vi "UpdateHawkeyeList.vi"(7 "WorkSpace / Repo path":path, 8 "error in (no error)":errorcluster, 10 "Library/Class Name":string, 11 "Config Refnum in":T1) -> (0 "error out":errorcluster, 1 "Indirect Dependency []":string[](array[string]), 2 "Direct Dependency []":string[](array[string]), 3 "Config Refnum out":T1)   [LabVIEW 2019, in "Hawkeye.lvlib"]
uses:
  Hawkeye.lvlib
  <vilib>/Utility/config.llb/Config Data RefNum.ctl
  <vilib>/Utility/config.llb/Write Key (String).vi
  <vilib>/Utility/config.llb/NI_LVConfig.lvlib
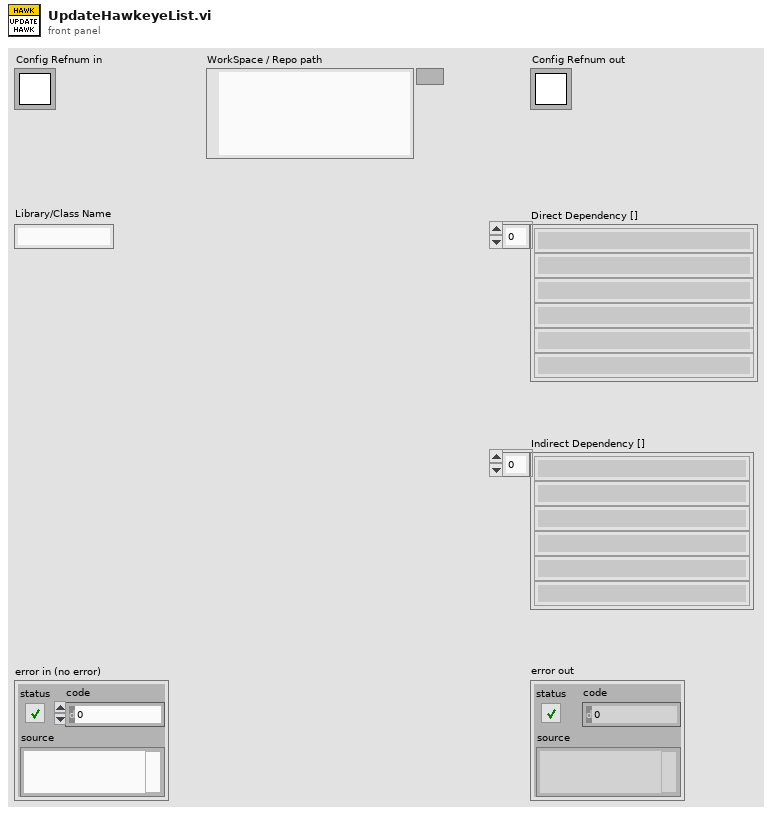
[diagram p1: front panel]
types:
  T1 = typedef "NI_LVConfig.lvlib/Config Data RefNum.ctl" = refnum<k1>
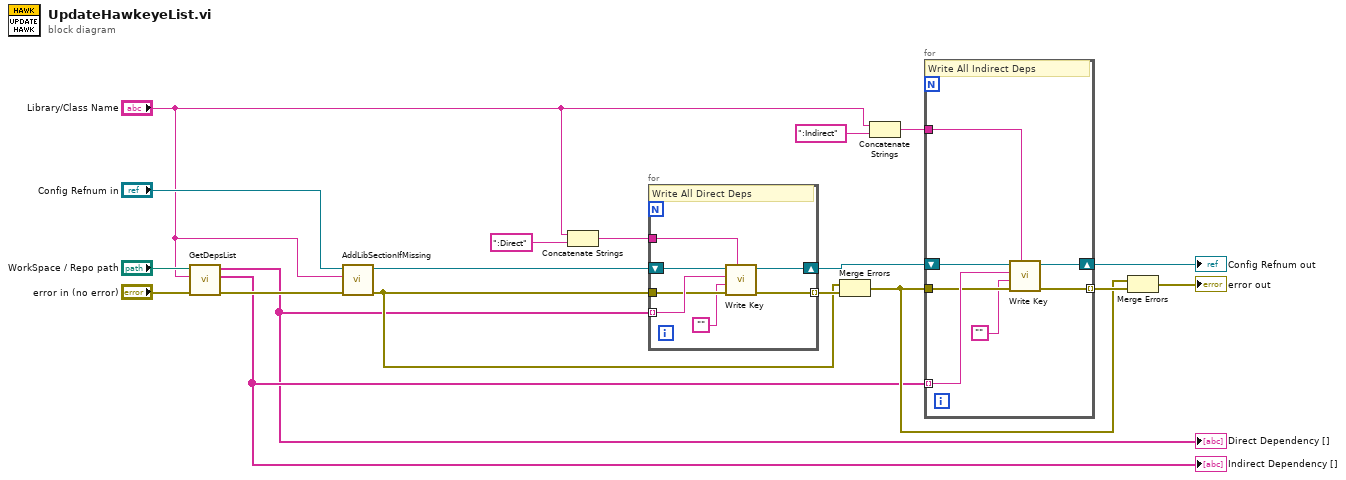
[diagram p0: block diagram]
diagram:
  n1 = call "GetDepsList.vi"("error in (no error)"="error in (no error)", "Library / Class Name"="Library/Class Name", "WorkSpace / Repo path"="WorkSpace / Repo path") -> ("error out"=w6:errorcluster, "Indirect Dependency []"=w2:string[], "Direct Dependency []"=w1:string[])  [unwired: 6 in]
  "Direct Dependency []" <- w1
  "Indirect Dependency []" <- w2
  n2 = call "AddLibSectionIfMissing.vi"("error in (no error)"=w6, "LibraryName"="Library/Class Name", "Config Refnum in"="Config Refnum in") -> ("error out"=w12:errorcluster, "Config Refnum out"=w14:T1)  [unwired: 7 in]
  n3 = Concatenate Strings("Library/Class Name", ":Direct" ("Type")) -> (w15:string)
  n4 = for {
    tunnel: w15 -> [w26]
    tunnel: w1 -> [w24] mode=indexing
    shift-right: [w23] -> w8
    shift-left: w14 -> [w25]
    tunnel: w12 -> [w22]
    tunnel: [w21] -> w13 mode=indexing
    # "Write All Direct Deps"
    n5 = call-poly <vilib>:"Write Key.vi"("section"=w26, "error in (no error)"=w22, "value"="", "key"=w24, "refnum"=w25) -> ("error out"=w21:errorcluster, "refnum out"=w23:T1)  [unwired: 4 in, 1 out]
  }
  n6 = Merge Errors(w12, w13) -> (w10:errorcluster)
  n7 = Concatenate Strings("Library/Class Name", ":Indirect" ("Type")) -> (w9:string)
  n8 = for {
    tunnel: w9 -> [w33]
    tunnel: w2 -> [w31] mode=indexing
    shift-right: [w30] -> w7
    shift-left: w8 -> [w32]
    tunnel: w10 -> [w29]
    tunnel: [w28] -> w11 mode=indexing
    # "Write All Indirect Deps"
    n9 = call-poly <vilib>:"Write Key.vi"("section"=w33, "error in (no error)"=w29, "value"="", "key"=w31, "refnum"=w32) -> ("error out"=w28:errorcluster, "refnum out"=w30:T1)  [unwired: 4 in, 1 out]
  }
  "Config Refnum out" <- w7
  n10 = Merge Errors(w10, w11) -> (→"error out":errorcluster)
